vi "Init.vi"(8 "error in (no error)":errorcluster, 11 "Data in":refnum<class "conc_SharedVar_Bool.lvclass">) -> (0 "error out":errorcluster, 3 "Data out":refnum<class "conc_SharedVar_Bool.lvclass">)   [LabVIEW 2021, in "conc_SharedVar_Bool.lvclass"]
uses:
  conc_SharedVar_Bool.lvclass
  conc_SharedVar_Bool.lvclass/conc_SharedVar_Bool.ctl
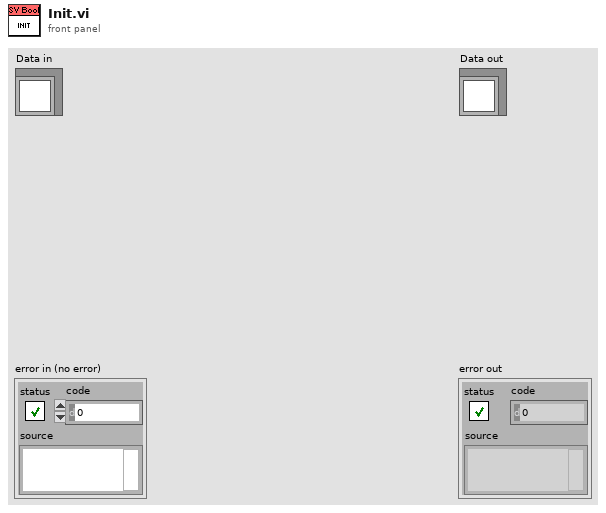
[diagram p1: front panel]
types:
  T1 = cluster{"Read Access":enum8{"Allowed", "Required", "None"}, "Write Access":enum8{"Allowed", "Required", "None"}}
  T2 = typedef "NI_Data Type.lvlib/Data Type.ctl" = enum8{"Invalid Type", "Void", "I8", "I16", "I32", "I64", "U8", "U16", "U32", "U64", "Single Float", "Double Float", "Extended Float", "Single Complex", "Double Complex", "Extended Complex", "Enum U8", "Enum U16", "Enum U32", "Enum U64", "Single Float With Unit", "Double Float With Unit", "Extended Float With Unit", "Single Complex with Unit", "Double Complex with Unit", "Extended Complex with Unit", "Boolean", "String", "Path", "Picture", "Tag", "Array", "Cluster", "Variant", "LV Variant", "Waveform", "Timestamp", "Digital Waveform", "Digital Data", "ExpressData", "Refnum", "External Data", "VI", "Poly VI", "LabVIEW Class Instance", "Fixed Point", "Set Collection", "Map Collection"}
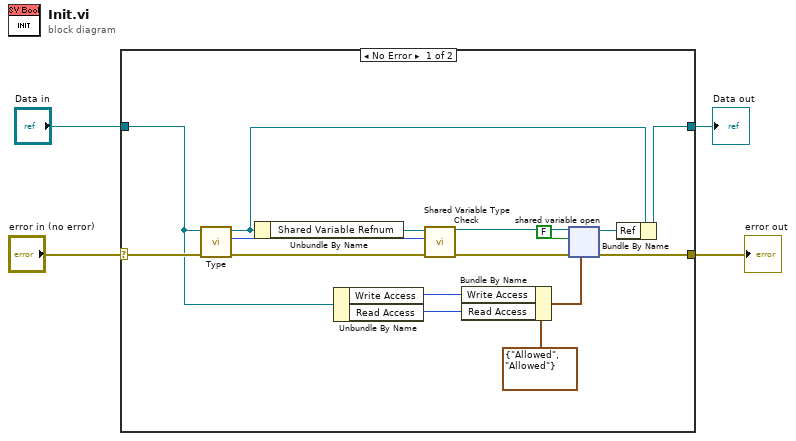
[diagram p0: block diagram]
diagram:
  n1 = case shown="No Error" "error in (no error)" {
    selector: "error in (no error)" -> [w18 w22]
    tunnel: [w20 w22] -> w4
    tunnel: [w19 w21] -> w3
    tunnel: "Data in" -> [w7 w21]
    frame No Error {
      n2 = call-dynamic "Type.vi"("error in (no error)"=w18, "Element in"=w7) -> ("error out"=w14:errorcluster, "Type"=w12:T2, "Element out"=w9:refnum<class "conc_SharedVar_Bool.lvclass">)  [unwired: 7 in]
      n3 = Unbundle By Name(w9) -> ("Shared Variable Refnum"=w8:refnum<k21>)
      n4 = Unbundle By Name(w7) -> ("Write Access"=w6:enum8{"Allowed", "Required", "None"}, "Read Access"=w5:enum8{"Allowed", "Required", "None"})
      n5 = call "Shared Variable Type Check.vi"("error in (no error)"=w14, "Type"=w12, "Shared Var in"=w8) -> ("error out"=w13:errorcluster, "Shared Var out"=w15:refnum<k21>)  [unwired: 6 in, 1 out]
      n6 = Bundle By Name(cluster=T1 {"Read Access"=enum."Allowed", "Write Access"=enum."Allowed"} ("access"), "Write Access"=w6, "Read Access"=w5) -> (w16:T1)
      n7 = shared-variable-open(w15, w13, FALSE, w16) -> (w10:refnum<k21>, w20:errorcluster)
      n8 = Bundle By Name(cluster=w9, "Ref"=w10) -> (w19:refnum<class "conc_SharedVar_Bool.lvclass">)
    }
    frame Error {
    }
  }
  "error out" <- w4
  "Data out" <- w3
